vi "Attenuator Pluck Data for Display.vi"(8 "Measurement Values":T1, 9 "Peak Variance (dB)":refnum<vi>, 10 "Frequency":refnum<vi>, 11 "Attenuation Variance":refnum<vi>) -> ()   [LabVIEW 2011]
uses:
  TypeDefs/Attenuator Measurement Values.ctl
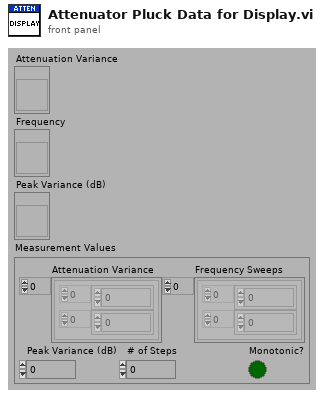
[diagram p1: front panel]
types:
  T1 = typedef "Attenuator Measurement Values.ctl" = cluster{"# of Steps":i32, "Attenuation Variance":cluster{"X":dbl[], "Y":dbl[]}[], "Frequency Sweeps":cluster{"X":dbl[], "Y":dbl[]}[], "Peak Variance (dB)":dbl, "Monotonic?":bool}
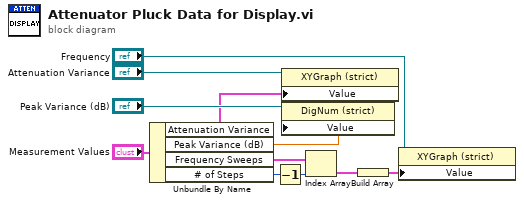
[diagram p0: block diagram]
diagram:
  n1 = Unbundle By Name("Measurement Values") -> ("Attenuation Variance"=w8:cluster{"X":dbl[], "Y":dbl[]}[], "Peak Variance (dB)"=w7:dbl, "Frequency Sweeps"=w6:cluster{"X":dbl[], "Y":dbl[]}[], "# of Steps"=w5:i32)
  n2 = Decrement(x=w5) -> (x-1=w4:i32)
  n3 = property class="XYGraph (strict)"(reference="Attenuation Variance", "Value"=w8) -> ()  [unwired: 1 in, 2 out]
  n4 = property class="DigNum (strict)"(reference="Peak Variance (dB)", "Value"=w7) -> ()  [unwired: 1 in, 2 out]
  n5 = Index Array(array=w6, index=w4) -> (element=w1:cluster{"X":dbl[], "Y":dbl[]})
  n6 = Build Array(w1) -> (w2:cluster{"X":dbl[], "Y":dbl[]}[])
  n7 = property class="XYGraph (strict)"(reference="Frequency", "Value"=w2) -> ()  [unwired: 1 in, 2 out]
